vi "DiffDrvOdom2_Update.vi"(8 "Right Distance M":dbl, 9 "Left Distance M":dbl, 10 "Gyro Reading":T4={"VALUE"=0.0, "COS"=1.0, "SIN"=0.0} {"SIN" format="%13.4f"; "COS" format="%13.4f"; "VALUE" format="%13.4f"}, 11 "In DIFF_DRIVE_ODOM":T1={"M_POSE_Meters"={"TRANSLATION"={"X"=0.0, "Y"=0.0}, "ROTATION"={"VALUE"=0.0, "COS"=1.0, "SIN"=0.0}}, "M_GyroOffset"={"VALUE"=0.0, "COS"=1.0, "SIN"=0.0}, "M_PrevAngle"={"VALUE"=0.0, "COS"=1.0, "SIN"=0.0}, "M_PrevLeftDist_M"=0.0, "M_PrevRightDist_M"=0.0, "M_InitLeftDist_M"=0.0, "M_InitRightDist_M"=0.0} {"M_PrevAngle"."SIN" format="%13.4f"; "M_PrevAngle"."COS" format="%13.4f"; "M_PrevAngle"."VALUE" format="%13.4f"; "M_GyroOffset"."SIN" format="%13.4f"; "M_GyroOffset"."COS" format="%13.4f"; "M_GyroOffset"."VALUE" format="%13.4f"; "M_POSE_Meters"."ROTATION"."SIN" format="%13.4f"; "M_POSE_Meters"."ROTATION"."COS" format="%13.4f"; "M_POSE_Meters"."ROTATION"."VALUE" format="%13.4f"; "M_POSE_Meters"."TRANSLATION"."Y" format="%14.3f"; "M_POSE_Meters"."TRANSLATION"."X" format="%14.3f"}) -> (1 "Pose Meters":T2={"TRANSLATION"={"X"=0.0, "Y"=0.0}, "ROTATION"={"VALUE"=0.0, "COS"=1.0, "SIN"=0.0}} {"ROTATION"."SIN" format="%13.4f"; "ROTATION"."COS" format="%13.4f"; "ROTATION"."VALUE" format="%13.4f"; "TRANSLATION"."Y" format="%14.3f"; "TRANSLATION"."X" format="%14.3f"}, 3 "Out DIFF_DRIVE_ODOM":T1={"M_POSE_Meters"={"TRANSLATION"={"X"=0.0, "Y"=0.0}, "ROTATION"={"VALUE"=0.0, "COS"=1.0, "SIN"=0.0}}, "M_GyroOffset"={"VALUE"=0.0, "COS"=1.0, "SIN"=0.0}, "M_PrevAngle"={"VALUE"=0.0, "COS"=1.0, "SIN"=0.0}, "M_PrevLeftDist_M"=0.0, "M_PrevRightDist_M"=0.0, "M_InitLeftDist_M"=0.0, "M_InitRightDist_M"=0.0} {"M_PrevAngle"."SIN" format="%13.4f"; "M_PrevAngle"."COS" format="%13.4f"; "M_PrevAngle"."VALUE" format="%13.4f"; "M_GyroOffset"."SIN" format="%13.4f"; "M_GyroOffset"."COS" format="%13.4f"; "M_GyroOffset"."VALUE" format="%13.4f"; "M_POSE_Meters"."ROTATION"."SIN" format="%13.4f"; "M_POSE_Meters"."ROTATION"."COS" format="%13.4f"; "M_POSE_Meters"."ROTATION"."VALUE" format="%13.4f"; "M_POSE_Meters"."TRANSLATION"."Y" format="%14.3f"; "M_POSE_Meters"."TRANSLATION"."X" format="%14.3f"})   [LabVIEW 2019, in "Trajectory_Library.lvlib"]
doc: "Updates the robot position on the field using distance measurements from encoders. This method is more numerically accurate than using velocities to integrate the pose and is also advantageous for teams that are using lower CPR encoders.\n \nInputs:\n - in_DiffDriveOdom -- DiffDriveOdom2 -- Diff Drive odometry data cluster\n - gyroAngle -- Rotation2d -- The angle reported by the gyroscope.\n - leftDistanceMeters -- Double -- The distance traveled by the left encoder.\n - rightDistanceMeters -- Double -- The distance traveled by the right encoder.\n\nOutputs:\n - out_DiffDriveOdom -- DiffDriveOdom2 -- Updated data cluster\n - pose -- Pose2d -- The new pose of the robot."
uses:
  Trajectory_Library.lvlib
  TypeDef/DIFF_DRIVE_ODOM2.ctl
  TypeDef/POSE2D.ctl
  TypeDef/TRANSLATION2D.ctl
  TypeDef/ROTATION2D.ctl
  Rotation2d_UnaryMinus.vi
  Rotation2d_RotateBy.vi
  Rotation2d_CreateAngle.vi
  Rotation2d_CreateXY.vi
  Util_CalcDist.vi
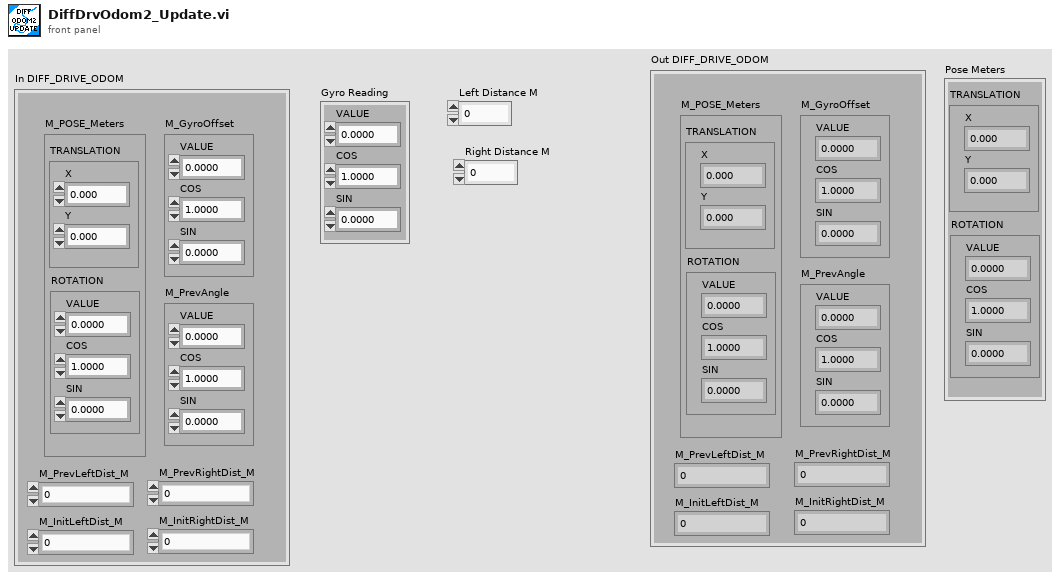
[diagram p1: front panel]
types:
  T1 = typedef "Trajectory_Library.lvlib/DIFF_DRIVE_ODOM2.ctl" = cluster{"M_POSE_Meters":T2, "M_GyroOffset":T4, "M_PrevAngle":T4, "M_PrevLeftDist_M":dbl, "M_PrevRightDist_M":dbl, "M_InitLeftDist_M":dbl, "M_InitRightDist_M":dbl}
  T2 = typedef "Trajectory_Library.lvlib/POSE2D.ctl" = cluster{"TRANSLATION":T3, "ROTATION":T4}
  T3 = typedef "Trajectory_Library.lvlib/TRANSLATION2D.ctl" = cluster{"X":dbl, "Y":dbl}
  T4 = typedef "Trajectory_Library.lvlib/ROTATION2D.ctl" = cluster{"VALUE":dbl, "COS":dbl, "SIN":dbl}
  T5 = typedef "Trajectory_Library.lvlib/TWIST2D.ctl" = cluster{"dX":dbl, "dY":dbl, "dTHETA":dbl}
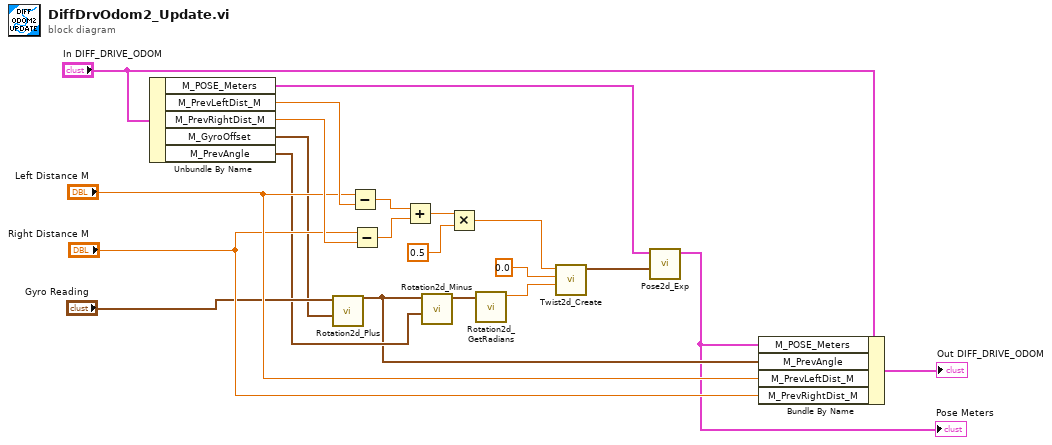
[diagram p0: block diagram]
diagram:
  n1 = Unbundle By Name("In DIFF_DRIVE_ODOM") -> ("M_POSE_Meters"=w3:T2, "M_PrevLeftDist_M"=w19:dbl, "M_PrevRightDist_M"=w18:dbl, "M_GyroOffset"=w10:T4, "M_PrevAngle"=w7:T4)
  n2 = call "Rotation2d_Plus.vi"("other ROTATION"=w10, "in ROTATION"="Gyro Reading") -> ("out ROTATION"=w4:T4)  [unwired: 9 in]
  n3 = Subtract(x="Left Distance M", y=w19) -> (x-y=w17:dbl)
  n4 = Subtract(x="Right Distance M", y=w18) -> (x-y=w16:dbl)
  n5 = Add(x=w17, y=w16) -> (x+y=w15:dbl)
  n6 = call "Rotation2d_Minus.vi"("other ROTATION"=w7, "in ROTATION"=w4) -> ("out ROTATION"=w6:T4)  [unwired: 9 in]
  n7 = Multiply(x=w15, y=0.5) -> (x*y=w9:dbl)
  n8 = call "Rotation2d_GetRadians.vi"("in ROTATION"=w6) -> ("AngleRadians"=w5:dbl)  [unwired: 10 in]
  n9 = call "Twist2d_Create.vi"("dTHETA"=w5, "dY"=0.0, "dX"=w9) -> ("TWIST"=w2:T5)  [unwired: 8 in]
  n10 = call "Pose2d_Exp.vi"("TWIST"=w2, "POSE"=w3) -> ("UpdatedPose"=w1:T2)  [unwired: 9 in]
  "Pose Meters" <- w1
  n11 = Bundle By Name(cluster="In DIFF_DRIVE_ODOM", "M_POSE_Meters"=w1, "M_PrevAngle"=w4, "M_PrevLeftDist_M"="Left Distance M", "M_PrevRightDist_M"="Right Distance M") -> (→"Out DIFF_DRIVE_ODOM":T1)
